vi "Quantile-Quantile Plot.vi"(10 "Data array 2":dbl[](array[numeric]) format="%#.6g", 11 "Data array 1":dbl[](array[numeric]) format="%#.6g") -> (3 "Quantile-Quantile Plot":cluster{dbl[], dbl[]}[](graph))   [LabVIEW 2023]
doc: "Computes the quantile-quantile plot of the data."
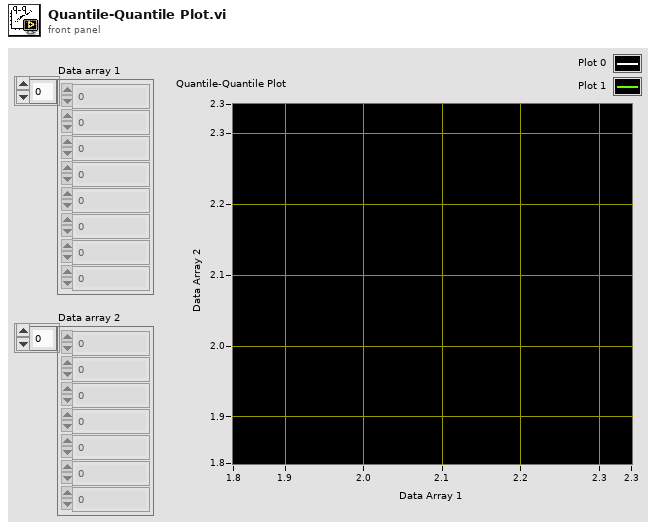
[diagram p1: front panel]
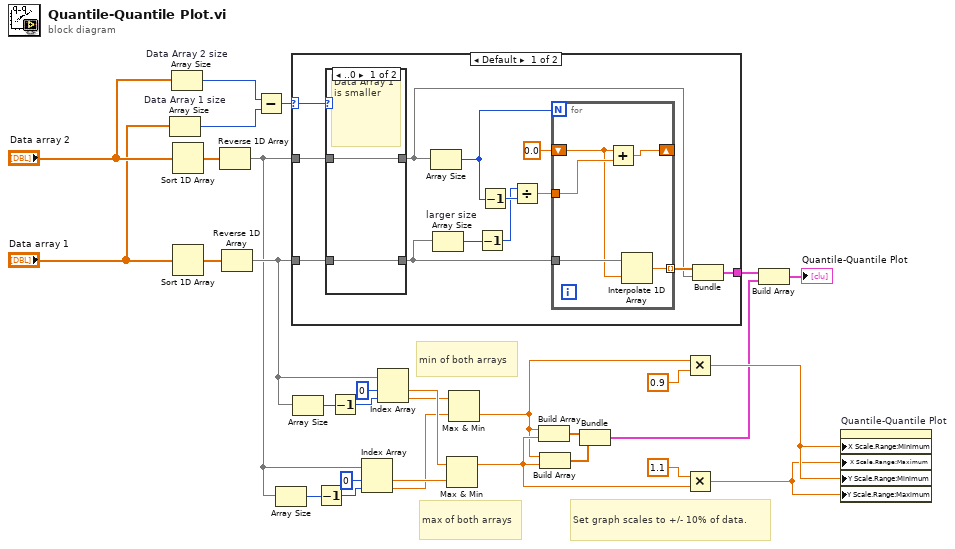
[diagram p0: block diagram]
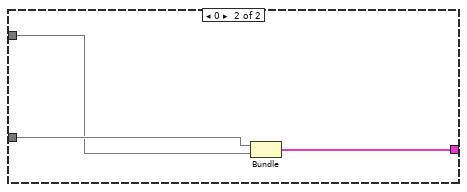
[diagram p3: hidden frame]
diagram:
  # "Set graph scales to +/- 10% of data."
  # "max of both arrays"
  # "min of both arrays"
  n1 = Array Size "Data Array 1 size"(array="Data array 1") -> (size(s)=w25:i32)
  n2 = Array Size "Data Array 2 size"(array="Data array 2") -> (size(s)=w26:i32)
  n3 = Sort 1D Array(array="Data array 2") -> (sorted array=w30:dbl[])
  n4 = Sort 1D Array(array="Data array 1") -> (sorted array=w28:dbl[])
  n5 = Reverse 1D Array(array=w30) -> (reversed array=w20:dbl[])
  n6 = Reverse 1D Array(array=w28) -> (reversed array=w24:dbl[])
  n7 = Subtract(x=w26, y=w25) -> (x-y=w3:i32)
  n8 = Array Size(array=w20) -> (size(s)=w13:i32)
  n9 = case shown="Default" w3 {
    selector: w3 -> [w32 _]
    tunnel: w20 -> [w43 w53]
    tunnel: w24 -> [w42 w54]
    tunnel: [w33 w55] -> w19
    frame Default {
      n10 = case shown="..0" w32 {
        tunnel: [w50 w52] -> w34
        tunnel: w43 -> [w50 w51]
        tunnel: [w49 w51] -> w38
        tunnel: w42 -> [w49 w52]
        frame ..0 {
          # "Data Array 1 is smaller"
        }
        frame 1.. {
          # "Data Array 2 is smaller"
        }
      }
      n11 = Array Size ("smaller size")(array=w34) -> (size(s)=w40:i32)
      n12 = Array Size "larger size"(array=w38) -> (size(s)=w41:i32)
      n13 = Decrement(x=w41) -> (x-1=w36:i32)
      n14 = Decrement(x=w40) -> (x-1=w37:i32)
      n15 = Divide(x=w36, y=w37) -> (x/y=w39:dbl)
      n16 = for {
        N: w40 -> [_]
        shift-right: [w46] -> _
        shift-left: 0.0 -> [w45]
        tunnel: w39 -> [w47]
        tunnel: w38 -> [w48]
        tunnel: [w44] -> w35 mode=indexing
        n17 = Add(x=w45, y=w47) -> (x+y=w46:dbl)
        n18 = Interpolate 1D Array(1:w45, 2:w48) -> (0:w44:dbl)
      }
      n19 = Bundle(w35, w34) -> (w33:cluster{dbl[], dbl[]})  [unwired: 1 in]
    }
    frame 0 {
      n20 = Bundle(w54, w53) -> (w55:cluster{dbl[], dbl[]})  [unwired: 1 in]
    }
  }
  n21 = Array Size(array=w24) -> (size(s)=w23:i32)
  n22 = Decrement(x=w13) -> (x-1=w14:i32)
  n23 = Decrement(x=w23) -> (x-1=w15:i32)
  n24 = Index Array(array=w20, index #1=0 ("index"), index #2=w14) -> (element #1=w10:dbl, element #2=w9:dbl)
  n25 = Index Array(array=w24, index #1=0 ("index"), index #2=w15) -> (element #1=w12:dbl, element #2=w11:dbl)
  n26 = Max & Min(x=w12, y=w10) -> (max(x,y)=w6:dbl)  [unwired: 1 out]
  n27 = Max & Min(x=w11, y=w9) -> (min(x,y)=w5:dbl)  [unwired: 1 out]
  n28 = Build Array(w5, w6) -> (w17:dbl[])
  n29 = Build Array(w5, w6) -> (w16:dbl[])
  n30 = Bundle(w17, w16) -> (w4:cluster{dbl[], dbl[]})  [unwired: 1 in]
  n31 = Multiply(x=w5, y=0.9) -> (x*y=w8:dbl)
  n32 = Multiply(x=1.1, y=w6) -> (x*y=w7:dbl)
  n33 = Build Array(w19, w4) -> (→"Quantile-Quantile Plot":cluster{dbl[], dbl[]}[])
  n34 = property on="Quantile-Quantile Plot" class="XYGraph (strict)"("X Scale.Range:Minimum"=w8, "X Scale.Range:Maximum"=w7, "Y Scale.Range:Minimum"=w8, "Y Scale.Range:Maximum"=w7) -> ()  [unwired: 2 in, 2 out]
